vi "AddLight.vi"(5 "Light State":enum16{"Inherit Value", "Off", "On"}(ring), 7 "At Infinity":bool, 8 "error in (no error)":errorcluster, 9 "Position":T1, 10 "Light Number":i32, 11 "3D Object in":refnum<class "3D Object.lvclass">) -> (0 "error out":errorcluster, 3 "3D Object out":refnum<class "3D Object.lvclass">)   [LabVIEW 2015, in "3D Object.lvclass"]
uses:
  3D Object.lvclass
  <vilib>/Utility/miscctls.llb/LV3DPointTypeDef.ctl
  3D Object.lvclass/3D Object.ctl
  <vilib>/picture/3D Picture Control/Helpers/Set Light (no reference).vi
  <vilib>/picture/3D Picture Control/NI_3D Picture Control.lvlib
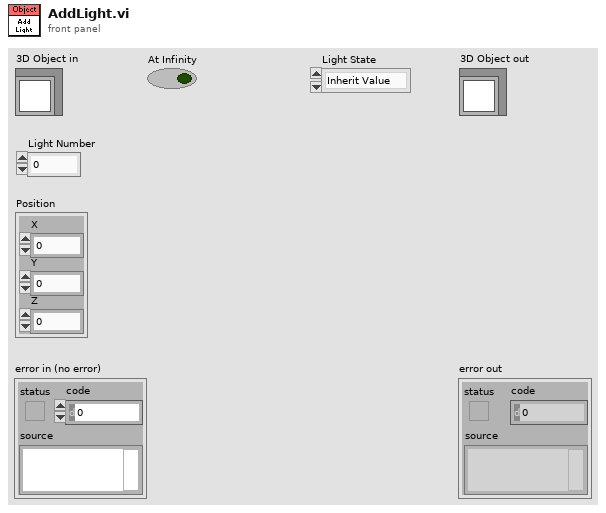
[diagram p1: front panel]
types:
  T1 = typedef "LV3DPointTypeDef.ctl" = cluster{"X":sgl, "Y":sgl, "Z":sgl}
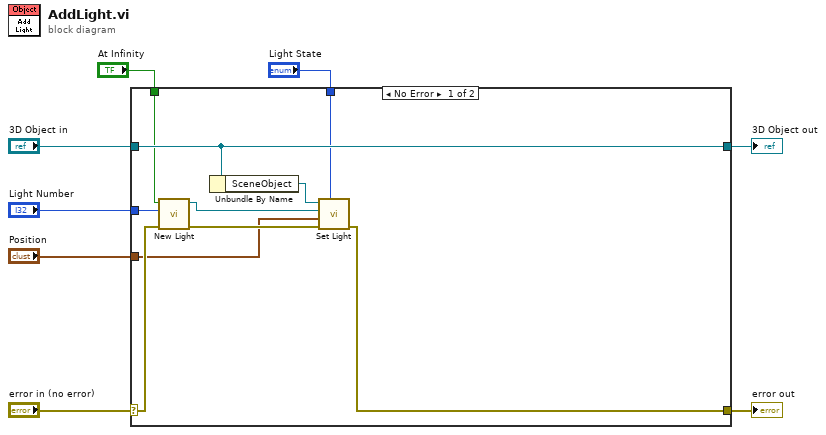
[diagram p0: block diagram]
diagram:
  n1 = case shown="No Error" "error in (no error)" {
    selector: "error in (no error)" -> [w14 w20]
    tunnel: [w12 w20] -> w7
    tunnel: [w18 w19] -> w5
    tunnel: "3D Object in" -> [w18 w19]
    tunnel: "At Infinity" -> [w15 _]
    tunnel: "Light Number" -> [w11 _]
    tunnel: "Position" -> [w10 _]
    tunnel: "Light State" -> [w9 _]
    frame No Error {
      n2 = call <vilib>:"New Light.vi"("error in (no error)"=w14, "Light Number"=w11, "At Infinity"=w15) -> ("error out"=w13:errorcluster, "New Light Refnum"=w16:refnum<vi>)  [unwired: 7 in]
      n3 = Unbundle By Name(w18) -> ("SceneObject"=w17:refnum<vi>)
      n4 = call-poly <vilib>:"Set Light.vi"("Light State"=w9, "error in (no error)"=w13, "Position"=w10, "Light Refnum In"=w16, "Scene Object In"=w17) -> ("error out"=w12:errorcluster)  [unwired: 5 in, 1 out]
    }
    frame Error {
    }
  }
  "error out" <- w7
  "3D Object out" <- w5
